vi "spawn_connection_handler.vi"(6 "Log Service":refnum<data-value>, 8 "error in (no error)":errorcluster, 10 "Connection":refnum<class "Connection.lvclass">, 11 "Connection Hanlder":refnum<class "Connection Handler.lvclass">) -> ()   [LabVIEW 2019, in "Socket API.lvlib" / "Socket Server.lvclass"]
uses:
  Socket Server.lvclass
  Connection Handler/Connection Handler.lvclass
  Connection/Connection.lvclass
  Utility API/Log Service/Log Service.lvclass
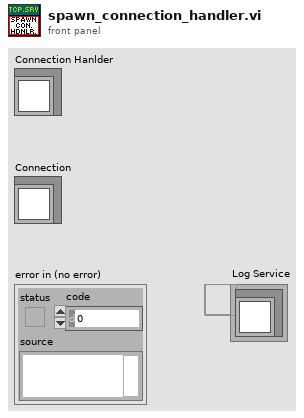
[diagram p1: front panel]
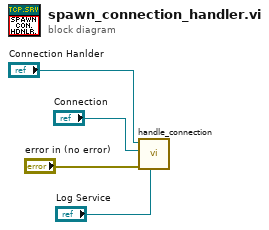
[diagram p0: block diagram]
diagram:
  n1 = call-dynamic "handle_connection.vi"("Log Service"="Log Service", "error in (no error)"="error in (no error)", "connection"="Connection", "Connection Handler in"="Connection Hanlder") -> ()  [unwired: 7 in, 1 out]
